vi "ReadTriggerNode.vi"(8 "Error In":errorcluster, 11 "Keithley2602 Node In":refnum<k20>) -> (0 "Error Out":errorcluster, 2 "Trigger Configuration":T1={"Input"={"Type"=enum."None", "Timeout (ms)"=0, "Delay (ms)"=0, "Digital IO Line (1-14)"=0, "Digital IO Mode"=enum."Falling"}, "Output"={"Type"=enum."None", "Delay (ms)"=0, "Digital IO Line (1-14)"=1, "Digital IO Mode"=enum."Falling", "Digital IO Pulse Width (sec)"=0.0}} {"Output"."Digital IO Line (1-14)" min=1 max=14 step=1}, 3 "Keithley2602 Node Out":refnum<k20>)   [LabVIEW 2012]
uses:
  TriggerConfiguration.ctl
  TriggerInputConfiguration.ctl
  TriggerInputType.ctl
  driver/Public/Controls/TriggerMode.ctl
  TriggerOutputConfiguration.ctl
  TriggerOutputType.ctl
  driver/Keithley-2602.lvlib
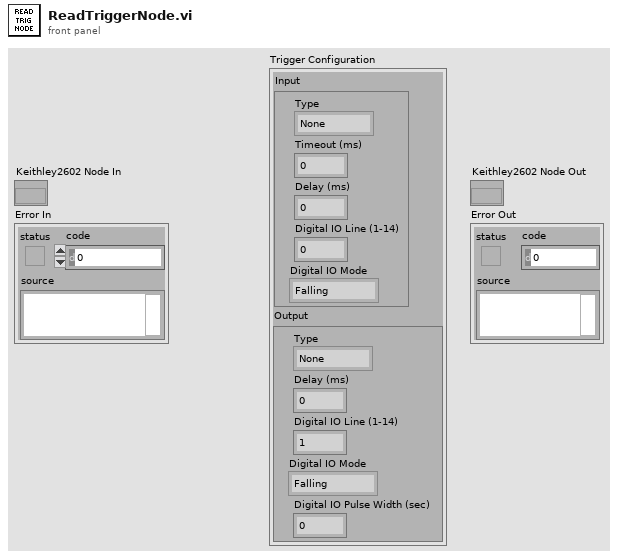
[diagram p1: front panel]
types:
  T1 = typedef "TriggerConfiguration.ctl" = cluster{"Input":T2, "Output":T5}
  T2 = typedef "TriggerInputConfiguration.ctl" = cluster{"Type":T3, "Timeout (ms)":u32, "Delay (ms)":u32, "Digital IO Line (1-14)":u8, "Digital IO Mode":T4}
  T3 = typedef "TriggerInputType.ctl" = enum16{"None", "Digital IO", "Bus"}
  T4 = typedef "Keithley-2602.lvlib/TriggerMode.ctl" = enum16{"Falling", "Rising", "Either", "Synchronous"}
  T5 = typedef "TriggerOutputConfiguration.ctl" = cluster{"Type":T6, "Delay (ms)":u32, "Digital IO Line (1-14)":u8, "Digital IO Mode":T4, "Digital IO Pulse Width (sec)":dbl}
  T6 = typedef "TriggerOutputType.ctl" = enum16{"None", "Digital IO", "Bus"}
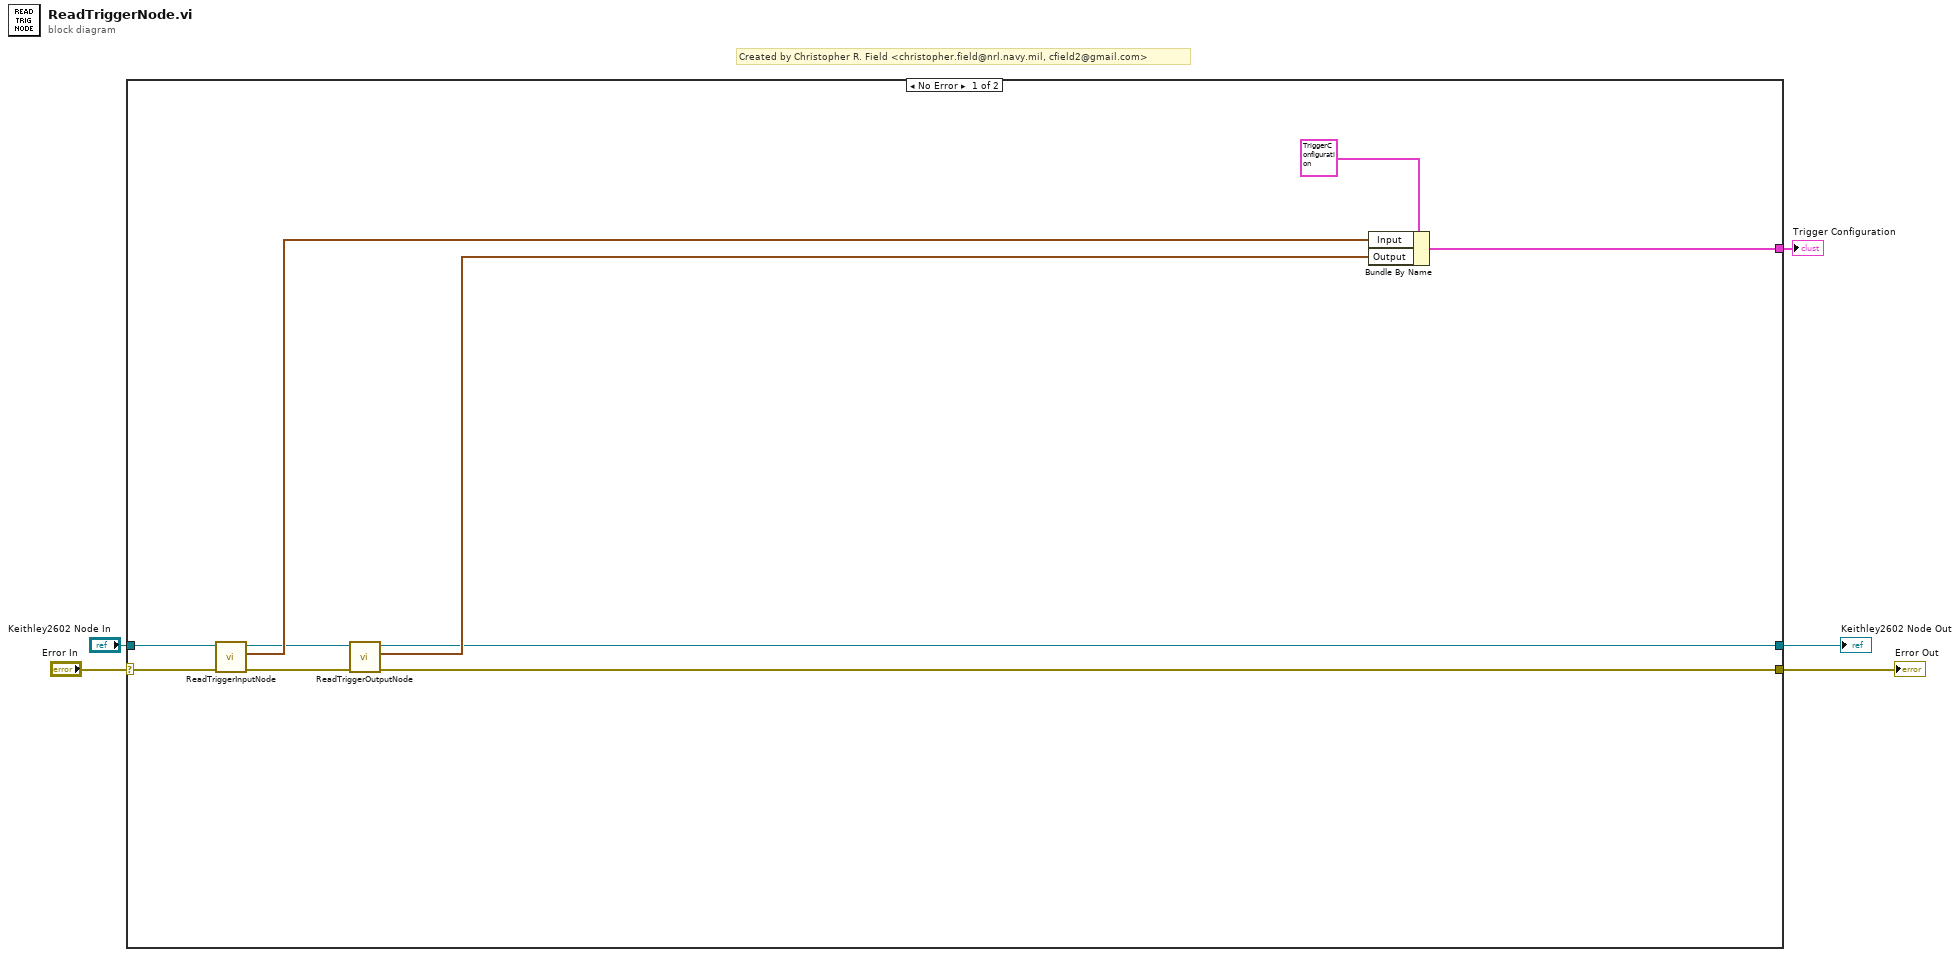
[diagram p0: block diagram]
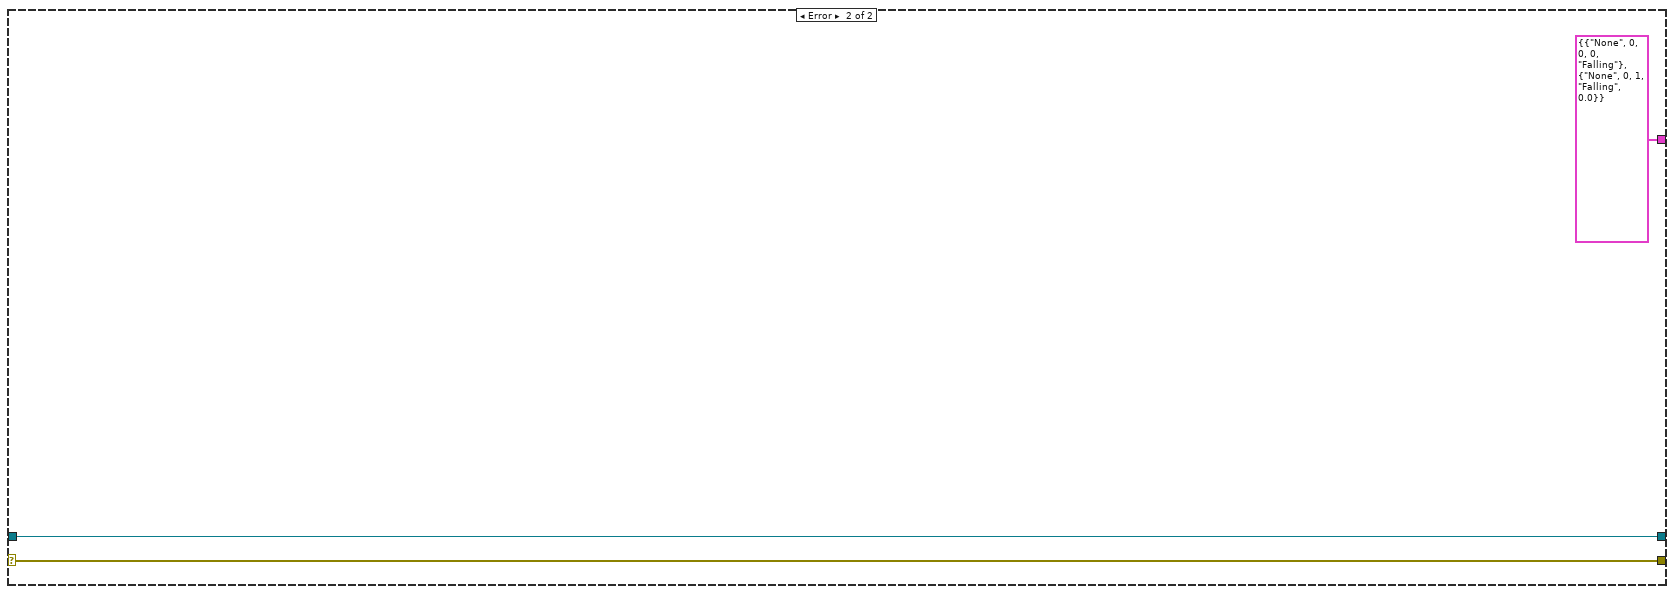
[diagram p2: hidden frame]
diagram:
  # "Created by Christopher R. Field <christopher.field@nrl.navy.mil, cfield2@gmail.com>"
  n1 = case shown="No Error" "Error In" {
    selector: "Error In" -> [w12 w17]
    tunnel: "Keithley2602 Node In" -> [w13 w18]
    tunnel: [w7 w18] -> w3
    tunnel: [w6 w17] -> w2
    tunnel: [w14 T1 {"Input"={"Type"=enum."None", "Timeout (ms)"=0, "Delay (ms)"=0, "Digital IO Line (1-14)"=0, "Digital IO Mode"=enum."Falling"}, "Output"={"Type"=enum."None", "Delay (ms)"=0, "Digital IO Line (1-14)"=1, "Digital IO Mode"=enum."Falling", "Digital IO Pulse Width (sec)"=0.0}} ("Trigger Configuration")] -> w1
    frame No Error {
      n2 = call "ReadTriggerInputNode.vi"("Error In"=w12, "Keithley2602 Node In"=w13) -> ("Error Out"=w9:errorcluster, "Trigger Input Configuration"=w11:T2, "Keithley2602 Node Out"=w10:refnum<k20>)  [unwired: 7 in]
      n3 = call "ReadTriggerOutputNode.vi"("Error In"=w9, "Keithley2602 Node In"=w10) -> ("Error Out"=w6:errorcluster, "Output Trigger Configuration"=w8:T5, "Keithley2602 Node Out"=w7:refnum<k20>)  [unwired: 7 in]
      n4 = Bundle By Name(cluster=T1 {"Input"={"Type"=enum."None", "Timeout (ms)"=0, "Delay (ms)"=0, "Digital IO Line (1-14)"=0, "Digital IO Mode"=enum."Falling"}, "Output"={"Type"=enum."None", "Delay (ms)"=0, "Digital IO Line (1-14)"=1, "Digital IO Mode"=enum."Falling", "Digital IO Pulse Width (sec)"=0.0}} ("Trigger Configuration"), "Input"=w11, "Output"=w8) -> (w14:T1)
    }
    frame Error {
    }
  }
  "Keithley2602 Node Out" <- w3
  "Error Out" <- w2
  "Trigger Configuration" <- w1
